vi "Test Logging.vi"(11 "Test Case In":refnum<class "File Sink.lvclass">) -> (0 "error out":errorcluster, 3 "Test Case Out":refnum<class "File Sink.lvclass">)   [LabVIEW 2020, in "File Sink.lvclass"]
uses:
  File Sink.lvclass
  File Sink.lvclass/File Sink.ctl
  4993e8ee-a06a-463a-9684-69129f64d5ce.vi
  <vilib>/Astemes/LUnit/Test Case.lvclass
  C:/Program Files (x86)/National Instruments/LabVIEW 2020/vi.lib/Astemes/LUnit/Test Case.lvclass
  C:/Program Files (x86)/National Instruments/LabVIEW 2020/vi.lib/Astemes/LUnit/LUnit Runnable.lvclass
  C:/Users/hughe_cx/Documents/05_repos/LVLog/Testing/File Sink/File Sink.lvclass
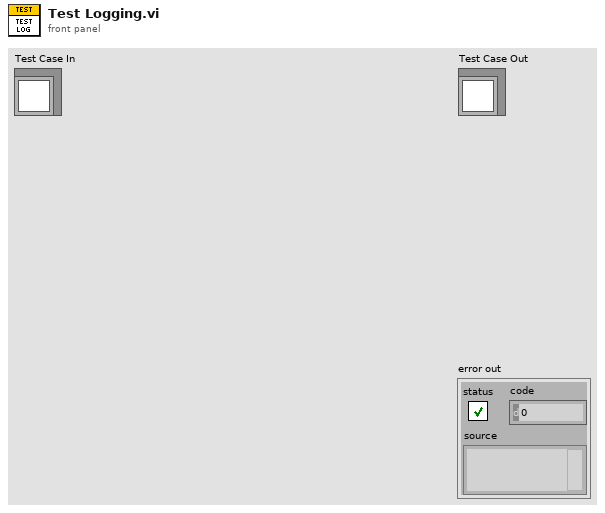
[diagram p1: front panel]
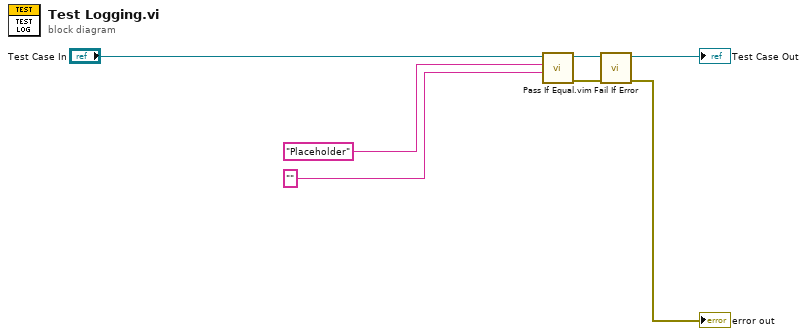
[diagram p0: block diagram]
diagram:
  n1 = call "Pass If Equal.vim"("Actual"="", "Expected"="Placeholder", "LUnit Test Case In"="Test Case In") -> ("error out"=w4:errorcluster, "LUnit Test Case Out"=w1:refnum<class "File Sink.lvclass">)  [unwired: 7 in]
  n2 = call <vilib>:"Fail If Error.vi"("error in (no error)"=w4, "LUnit Test Case In"=w1) -> ("error out"=→"error out":errorcluster, "LUnit Test Case Out"=→"Test Case Out":refnum<class "File Sink.lvclass">)  [unwired: 8 in]
